vi "ChangeDC.vi"(7 "LabVIEW Web Service Request":refnum<class "Web Request.lvclass">, 10 "blue":u8, 11 "dc":dbl) -> ()   [LabVIEW 2014]
uses:
  <vilib>/wsapi/Web Request.lvclass
  Controller/Controls/Enqueuer Enum.ctl
  CRDS/Actor Messages/Change Red DC MSG/Change Red DC MSG.lvclass
  CRDS/Actor Messages/Change Red DC MSG/Change Red DC MSG.lvclass/Change Red DC MSG.ctl
  CRDS/Actor Messages/Change Blue DC MSG/Change Blue DC MSG.lvclass
  CRDS/Actor Messages/Change Blue DC MSG/Change Blue DC MSG.lvclass/Change Blue DC MSG.ctl
  CRDS/Actor Messages/Change Red DC MSG/DC.vi
  CRDS/Actor Messages/Change Blue DC MSG/Write Rate (Hz).vi
  Controller/Controller.lvclass
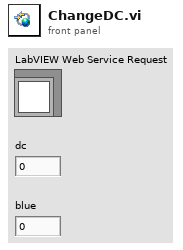
[diagram p1: front panel]
types:
  T1 = typedef "Controller.lvlib/Controller.lvclass/Enqueuer Enum.ctl" = enum8{"PAS", "CRDS", "File", "O3Lamp"}
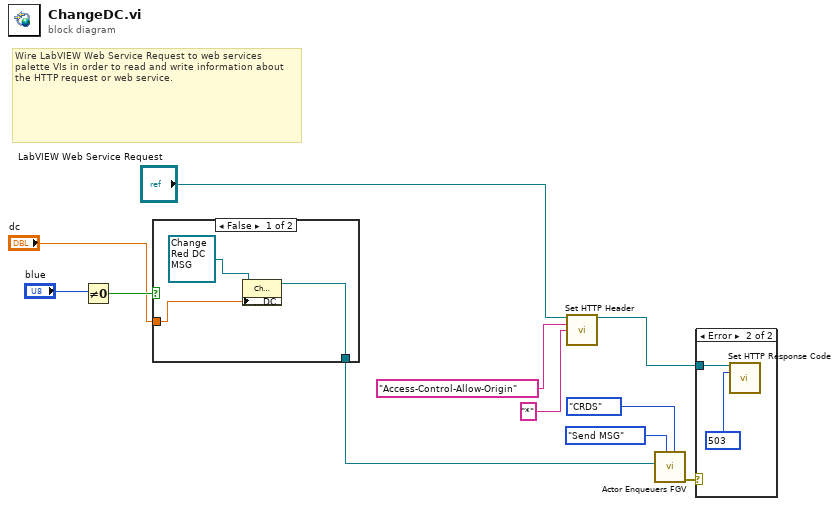
[diagram p0: block diagram]
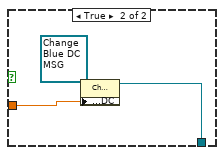
[diagram p2: hidden frame]
diagram:
  # "Wire LabVIEW Web Service Request to web services palette VIs in order to read and write information about the HTTP request or web service."
  n1 = Not Equal To 0?(x="blue") -> (x != 0?=w3:bool)
  n2 = case shown="False" w3 {
    tunnel: "dc" -> [w14 w16]
    tunnel: [w12 w15] -> w1
    frame False {
      n3 = property class="Change Red DC MSG"(reference=refnum<class "Change Red DC MSG.lvclass"> refnum ("eCRDS Library.lvlib:Change Blue MSG"), "Accessors:DC"=w14) -> (reference out=w12:refnum<class "Change Red DC MSG.lvclass">)  [unwired: 1 in, 1 out]
    }
    frame True {
      n4 = property class="Change Blue DC MSG"(reference=refnum<class "Change Blue DC MSG.lvclass"> refnum ("eCRDS Library.lvlib:Change Blue MSG"), "Accessors:DC"=w16) -> (reference out=w15:refnum<class "Change Blue DC MSG.lvclass">)  [unwired: 1 in, 1 out]
    }
  }
  n5 = call <vilib>:"Set HTTP Header.vi"("LabVIEW Web Service Request"="LabVIEW Web Service Request", "header"="Access-Control-Allow-Origin", "header value"="*") -> ("LabVIEW Web Service Request out"=w6:refnum<class "Web Request.lvclass">)  [unwired: 11 in, 1 out]
  n6 = call "Actor Enqueuers FGV.vi"("Enqueuer"=Enqueuer_Enum."CRDS", "State"=enum16{"Store", "Send MSG"}."Send MSG", "MSG"=w1) -> ("error out"=w9:errorcluster)  [unwired: 8 in]
  n7 = case shown="Error" w9 {
    tunnel: w6 -> [_ w19]
    frame No Error {
    }
    frame Error {
      w18 = 503 items=["100"=100, "101"=101, "200"=200, "201"=201, "202"=202, "203"=203, "204"=204, "205"=205, "206"=206, "300"=300, "301"=301, "302"=302, "303"=303, "304"=304, "305"=305, "306"=306, "307"=307, "400"=400, "401"=401, "402"=402, "403"=403, "404"=404, "405"=405, "406"=406, "407"=407, "408"=408, "409"=409, "410"=410, "411"=411, "412"=412, "413"=413, "414"=414, "415"=415, "416"=416, "417"=417, "500"=500, "501"=501, "502"=502, "503"=503, "504"=504, "505"=505] ("response code (200)")
      n8 = call <vilib>:"Set HTTP Response Code.vi"("LabVIEW Web Service Request"=w19, "response code (200)"=w18) -> ()  [unwired: 12 in, 2 out]
    }
  }
